vi "WeatherStation.vi"() -> ()   [LabVIEW 2020]
uses:
  Dane stacji pogodowej (cluster indicator).ctl
  strzalki.ctl
  <vilib>/Utility/file.llb/Write Delimited Spreadsheet (DBL).vi
panel:
  out "?":bool
  out "?":bool
  out "?":bool
  out "?":bool
  out "?":bool
  out "Opady":string
  out "Cluster":T1 {"Prędkość wiatru km/h" scale=0.0..80.0; "Opad [mm]" scale=0.0..50.0; "Temp.[°C]" scale=-5.0..40.0}
  out "Prędkość wiatru":string
  out "Temperatura":string
  out "Gołoledź":string
  in  "stop":bool
  # "Kontrolki ostrzegawcze"
  # "KIerunek wiatru"
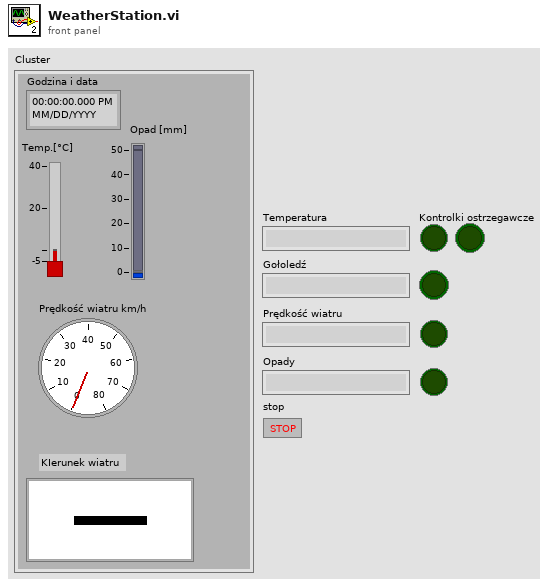
[diagram p1: front panel]
types:
  T1 = typedef "Dane stacji pogodowej (cluster indicator).ctl" = cluster{"Godzina i data":timestamp, "Temp.[°C] ":dbl, "Opad [mm]":dbl, "Prędkość wiatru km/h":dbl, "Ring":T2}
  T2 = typedef "strzalki.ctl" = u16
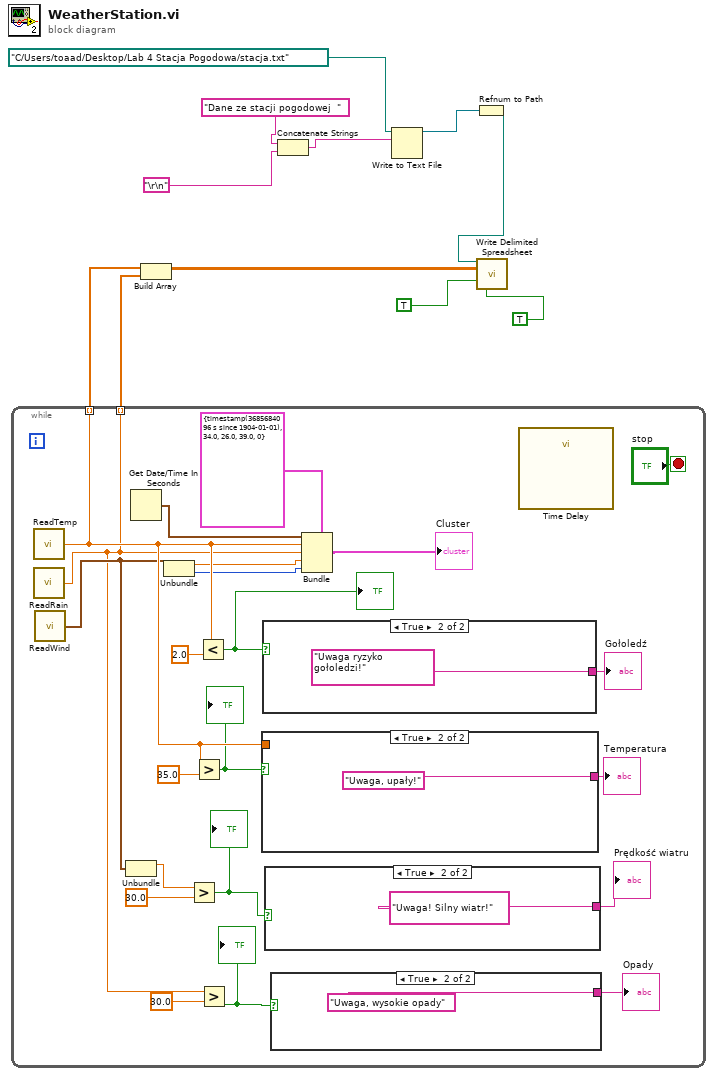
[diagram p0: block diagram]
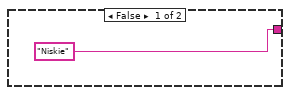
[diagram p2: hidden frame]
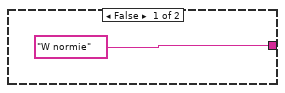
[diagram p3: hidden frame]
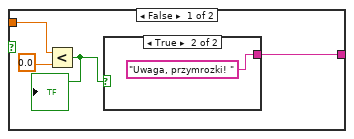
[diagram p4: hidden frame]
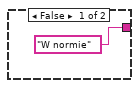
[diagram p5: hidden frame]
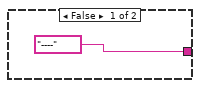
[diagram p6: hidden frame]
diagram:
  n1 = while {
    tunnel: [w25] -> w7 mode=indexing
    tunnel: [w12] -> w6 mode=indexing
    stop <- "stop" stop-if-true
    n2 = call "ReadTemp.vi"() -> ("Temperature, degC"=w25:dbl)
    n3 = call "ReadRain.vi"() -> ("Rain, mm"=w12:dbl)
    n4 = call "ReadWind.vi"() -> ("Wind Data"=w24:cluster{"Wind Speed":dbl, "Wind Direction":u16})
    n5 = Unbundle(w24) -> ("Wind Speed"=w28:dbl)  [unwired: 1 out]
    n6 = Get Date/Time In Seconds() -> (seconds since 1Jan1904=w19:timestamp)
    n7 = Unbundle(w24) -> ("Wind Speed"=w23:dbl, "Wind Direction"=w13:u16)
    n8 = Greater?(x=w28, y=30.0) -> (0:w15:bool)
    "?" <- w15
    n9 = Greater?(x=w25, y=35.0) -> (0:w16:bool)
    "?" <- w16
    n10 = Less?(x=w25, y=2.0) -> (x < y?=w17:bool)
    "?" <- w17
    n11 = Greater?(x=w12, y=30.0) -> (0:w14:bool)
    "?" <- w14
    n12 = case shown="True" w16 {
      tunnel: [w39 "Uwaga, upały!"] -> w30
      tunnel: w25 -> [w41 _]
      frame False {
        n13 = Less?(x=w41, y=0.0) -> (x < y?=w38:bool)
        "?" <- w38
        n14 = case shown="True" w38 {
          tunnel: ["W normie" "Uwaga, przymrozki! "] -> w39
          frame False {
          }
          frame True {
          }
        }
      }
      frame True {
      }
    }
    "Temperatura" <- w30
    n15 = case shown="True" w17 {
      tunnel: ["----" "Uwaga ryzyko gołoledzi!"] -> w32
      frame False {
      }
      frame True {
      }
    }
    "Gołoledź" <- w32
    n16 = case shown="True" w15 {
      tunnel: ["W normie" "Uwaga! Silny wiatr!"] -> w27
      frame False {
      }
      frame True {
      }
    }
    "Prędkość wiatru" <- w27
    n17 = case shown="True" w14 {
      tunnel: ["Niskie" "Uwaga, wysokie opady"] -> w20
      frame False {
      }
      frame True {
      }
    }
    "Opady" <- w20
    n18 = Bundle(cluster=T1 {"Godzina i data"=timestamp(3685684096.844536 s since 1904-01-01), "Temp.[°C] "=34.0, "Opad [mm]"=26.0, "Prędkość wiatru km/h"=39.0, "Ring"=0} ("Cluster"), "Godzina i data"=w19, "Temp.[°C]"=w25, "Opad [mm]"=w12, "Prędkość wiatru km/h"=w23, "Ring"=w13) -> (→"Cluster":T1)
    n19 = call "Time Delay"() -> ()  [unwired: 11 in, 1 out]
  }
  n20 = Build Array(w7, w6) -> (w4:dbl[][])
  n21 = Concatenate Strings("Dane ze stacji pogodowej  ", "\r\n") -> (w3:string)
  n22 = Write to Text File(file (use dialog)=path "C:/Users/toaad/Desktop/Lab 4 Stacja Pogodowa/stacja.txt" ("file path (dialog if empty)"), text=w3) -> (refnum out=w10:refnum<file>)  [unwired: 2 in, 2 out]
  n23 = Refnum to Path(1:w10) -> (0:w5:path)
  n24 = call-poly <vilib>:"Write Delimited Spreadsheet.vi"("file path (dialog if empty)"=w5, "2D data"=w4, "append to file? (new file:F)"=TRUE, "transpose? (no:F)"=TRUE) -> ()  [unwired: 10 in, 2 out]
